vi "Variant_To_DVR.vi"(8 "error in (no error)":errorcluster, 11 "Variant":variant) -> (0 "error out":errorcluster, 3 "DVR":refnum<data-value>)   [LabVIEW 2022 SP3, in "TopLevel.lvclass"]
uses:
  TopLevel.lvclass
  Typedefs/Private Data.ctl
  Typedefs/UserEvents.ctl
  Typedefs/API Event Data.ctl
  Typedefs/API Task State.ctl
  Motor Controller/Typedefs/Status_TopLevel--Cluster.ctl
  Common/Controls/TD MasterConfiguration DLPC2--cluster.ctl
  Common/Controls/DLPC2_Path--Cluster.ctl
  Common/Controls/TD HeadColorPaneMappingAll--cluster.ctl
  Common/Controls/TD HeadColorPaneMapping--cluster.ctl
  Typedefs/SpitVoltages--Cluster.ctl
  Typedefs/PrimingMode APIData.ctl
  Typedefs/PurgeMode--Enum.ctl
  Typedefs/PrinterHeads--Enum.ctl
  Common/Controls/GenericEventData--Cluster.ctl
  Typedefs/LoginEventData--CLuster.ctl
  Typedefs/UserLevel--Enum.ctl
  Motor Controller/Motor Controller.lvclass
  IO/IO.lvclass
  GIS Printer/GIS Printer.lvclass
  Typedefs/Digilens Config Cluster.ctl
  Typedefs/Motor Controller Config Data.ctl
  IO/Typedefs/IO Config Data.ctl
  IO/Typedefs/DCON_DeviceConfig--Cluster.ctl
  IO/Typedefs/Channel Data.ctl
  GIS Printer/Typedefs/PrinterConfiguration--Cluster.ctl
  DAQWFE/LV_Source/Subsystems/DAQ/DataTypes/TD DAQ Settings--cluster.ctl
  DAQWFE/LV_Source/Subsystems/DAQ/DataTypes/TD DI Instrument Settings--cluster.ctl
  DAQWFE/LV_Source/Subsystems/DAQ/DataTypes/TD AI Instrument Settings--cluster.ctl
  DAQWFE/LV_Source/Subsystems/DAQ/DataTypes/TD AI InstSettings--cluster.ctl
  DAQWFE/LV_Source/Subsystems/DAQ/Process/ProcessSupport/TD SimAI Ranges--cluster.ctl
  Database/Database.lvclass
  DLP2/DLP2.lvclass
  DAQWFE/LV_Source/Subsystems/DAQ/DAQ.lvclass
  <vilib>/TELLC/Dynamic CVT API/TD Dynamic CVT DVR--ref.ctl
  Common/Controls/DLPConfig_Initialization.ctl
  DLP2/DataTypes/DLP2_PrinterCompensationProperties.ctl
  DLP2/DataTypes/DLP2_PrinterHeadProperties.ctl
  Common/Controls/DLPConfig)Init_HeadPropertyAttr--Cluster.ctl
  DLP2/DataTypes/DLP2_PrinterMaterialProperties.ctl
  Typedefs/InkIdleNodeConfigXML--Cluster.ctl
  Typedefs/InkProcessNodeConfigXML--Cluster.ctl
  Common/Controls/PersistentData--Cluster.ctl
  Typedefs/processMode--enum.ctl
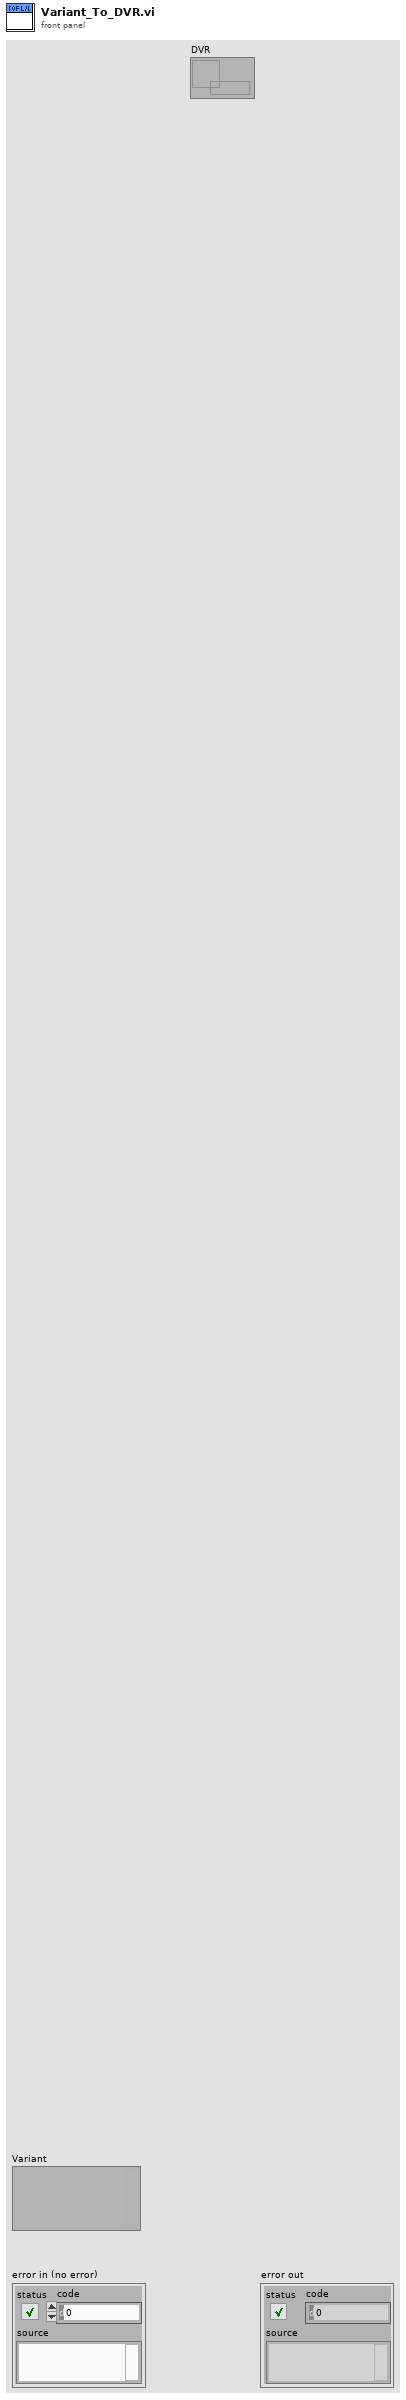
[diagram p1: front panel]
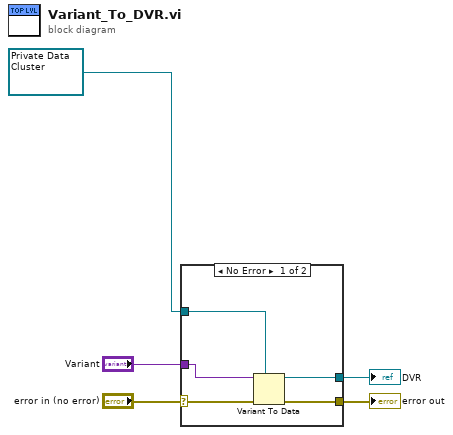
[diagram p0: block diagram]
diagram:
  n1 = case shown="No Error" "error in (no error)" {
    selector: "error in (no error)" -> [w10 w12]
    tunnel: [w9 w12] -> w4
    tunnel: "Variant" -> [w8 _]
    tunnel: [w7 w11] -> w1
    tunnel: refnum<data-value> refnum ("data value reference") -> [w6 w11]
    frame No Error {
      n2 = Variant To Data(error in=w10, type=w6, Variant=w8) -> (data=w7:refnum<data-value>, error out=w9:errorcluster)
    }
    frame Error {
    }
  }
  "error out" <- w4
  "DVR" <- w1
